vi "Decide if iteration successful.vi"(8 "error in (no error)":errorcluster, 11 "RSA in":refnum<class "RSA.lvclass">) -> (0 "error out":errorcluster, 3 "RSA out":refnum<class "RSA.lvclass">)   [LabVIEW 2012, in "RSA.lvclass"]
uses:
  RSA.lvclass
  RSA.lvclass/RSA.ctl
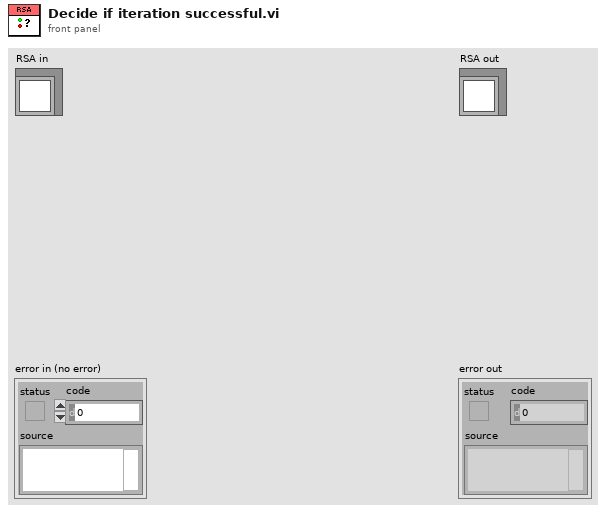
[diagram p1: front panel]
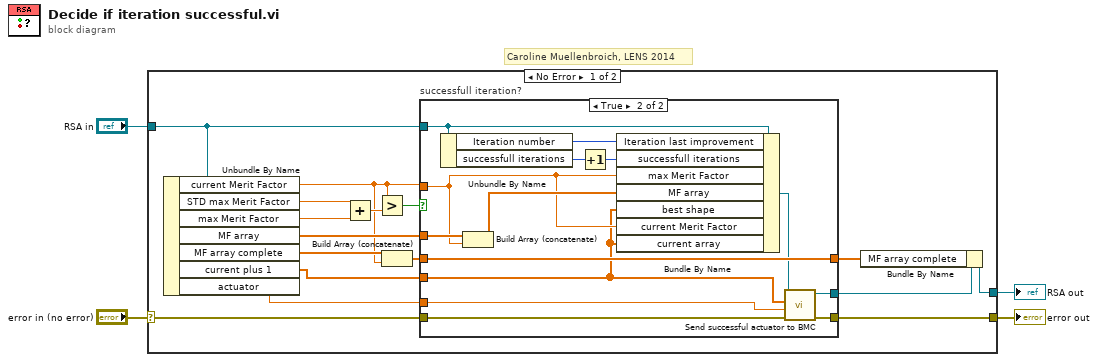
[diagram p0: block diagram]
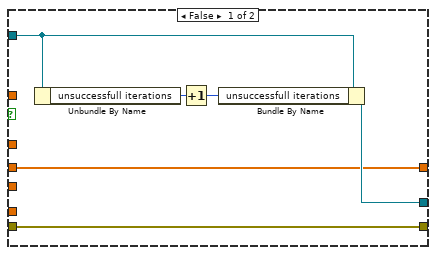
[diagram p2: hidden frame]
diagram:
  # "Caroline Muellenbroich, LENS 2014"
  n1 = case shown="No Error" "error in (no error)" {
    selector: "error in (no error)" -> [w12 w42]
    tunnel: [w9 w42] -> w3
    tunnel: [w16 w41] -> w1
    tunnel: "RSA in" -> [w17 w41]
    frame No Error {
      n2 = Unbundle By Name(w17) -> ("current Merit Factor"=w7:dbl, "STD max Merit Factor"=w20:dbl, "max Merit Factor"=w8:dbl, "MF array"=w14:dbl[], "MF array complete"=w13:dbl[], "current plus 1"=w6:dbl[], "actuator"=w5:dbl)
      n3 = Add(x=w20, y=w8) -> (x+y=w19:dbl)
      n4 = Greater?(x=w7, y=w19) -> (0:w18:bool)
      n5 = Build Array (concatenate)(w13, w7) -> (w11:dbl[])
      n6 = case "successfull iteration?" shown="True" w18 {
        tunnel: w17 -> [w24 w39]
        tunnel: [w23 w32] -> w15
        tunnel: w7 -> [_ w33]
        tunnel: w14 -> [_ w36]
        tunnel: w5 -> [_ w28]
        tunnel: w12 -> [w21 w29]
        tunnel: w11 -> [w22 w34]
        tunnel: [w22 w34] -> w10
        tunnel: [w21 w31] -> w9
        tunnel: w6 -> [_ w27]
        frame False {
          n7 = Unbundle By Name(w24) -> ("unsuccessfull iterations"=w26:i32)
          n8 = Increment(x=w26) -> (x+1=w25:i32)
          n9 = Bundle By Name(cluster=w24, "unsuccessfull iterations"=w25) -> (w23:refnum<class "RSA.lvclass">)
        }
        frame True {
          n10 = Unbundle By Name(w39) -> ("Iteration number"=w37:i32, "successfull iterations"=w40:i32)
          n11 = Build Array (concatenate)(w36, w33) -> (w35:dbl[])
          n12 = Increment(x=w40) -> (x+1=w38:i32)
          n13 = Bundle By Name(cluster=w39, "Iteration last improvement"=w37, "successfull iterations"=w38, "max Merit Factor"=w33, "MF array"=w35, "best shape"=w27, "current Merit Factor"=w33, "current array"=w27) -> (w30:refnum<class "RSA.lvclass">)
          n14 = call-dynamic "Send successful actuator to BMC.vi"("error in (no error)"=w29, "actuator in"=w28, "current plus 1 in"=w27, "RSA in"=w30) -> ("error out"=w31:errorcluster, "RSA out"=w32:refnum<class "RSA.lvclass">)  [unwired: 6 in]
        }
      }
      n15 = Bundle By Name(cluster=w15, "MF array complete"=w10) -> (w16:refnum<class "RSA.lvclass">)
    }
    frame Error {
    }
  }
  "error out" <- w3
  "RSA out" <- w1
